vi "JV Measurement.vi"(4 "Compliance (A)":dbl=0.01, 6 "Force Channel":u16(ring) items=["Channel A", "Channel B"], 8 "Delay (s)":dbl, 9 "Max (V)":dbl, 11 "Step (V)":dbl=0.1) -> ()   [LabVIEW 2011]
uses:
  <vilib>/Utility/file.llb/Write To Spreadsheet File (string).vi
  C:/Program Files (x86)/National Instruments/LabVIEW 2009/instr.lib/Keithley 2600 Series/Keithley 2600 Series.lvlib
panel:
  in  "Sample Name":string
  in  "Device Area (cm^2)":dbl=0.12
  out "XY Graph":cluster{dbl[], dbl[]}(graph)
  in  "Experiment Title":string
  in  "User Name":string
  in  "Stabilisation level \n(A or V depending on mode)":dbl=-1.6
  in  "Stabilisation time (ms)":dbl
  in  "Stabilisation mode":u16(ring) items=["Current", "Voltage"]
  in  "Max to min voltage sweep first?":bool
  in  "Min (V)":dbl=-1.6
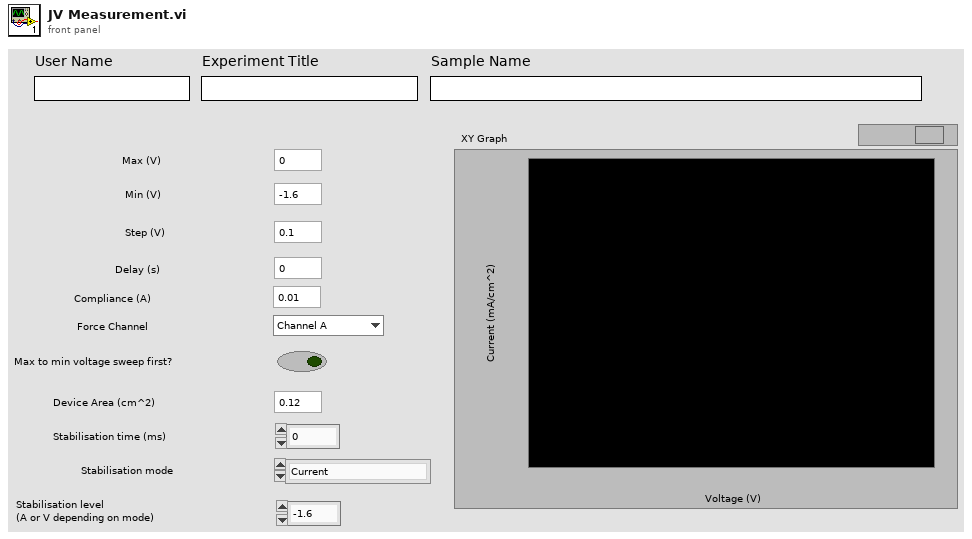
[diagram p1: front panel]
types:
  T1 = enum32{"Current", "Voltage", "IV", "Resistance", "Power"}
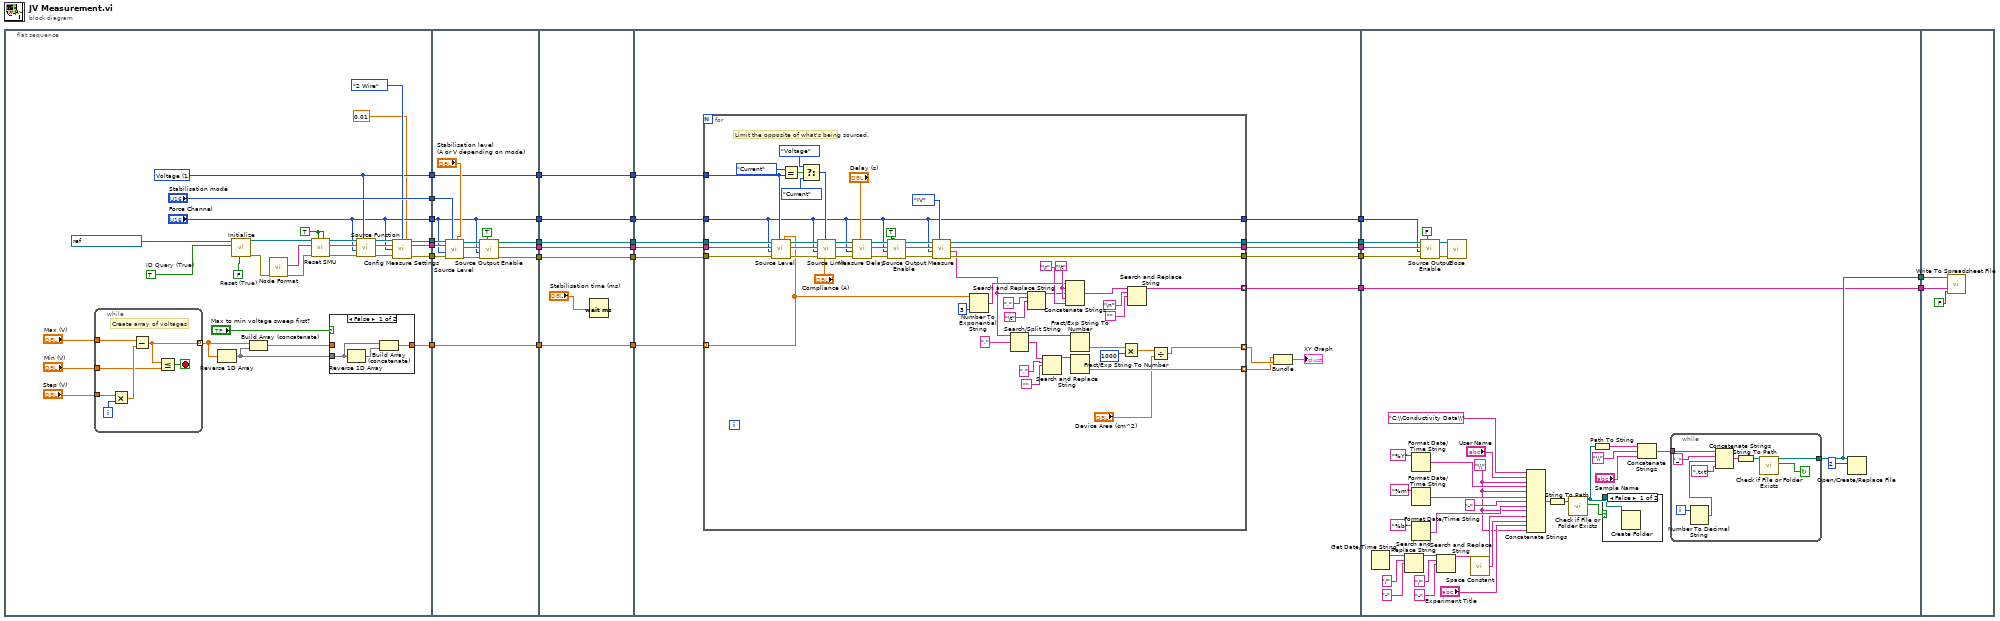
[diagram p0: block diagram]
diagram:
  n1 = flat-sequence {
    tunnel: [w29] -> w26
    tunnel: [w30] -> w25
    tunnel: ["Stabilisation mode"] -> w24
    tunnel: ["Force Channel"] -> w23
    tunnel: [w38] -> w22
    tunnel: [w37] -> w21
    tunnel: [w36] -> w20
    tunnel: w26 -> [w69]
    tunnel: w25 -> [w82]
    tunnel: w24 -> [w71]
    tunnel: w23 -> [w68]
    tunnel: w22 -> [w75]
    tunnel: w21 -> [w77]
    tunnel: w20 -> [w76]
    tunnel: [w82] -> w19
    tunnel: [w74] -> w16
    tunnel: [w73] -> w14
    tunnel: [w72] -> w12
    tunnel: [w69] -> w10
    tunnel: [w68] -> w8
    tunnel: w19 -> [w89]
    tunnel: [w89] -> w18
    tunnel: [w88] -> w17
    tunnel: w16 -> [w88]
    tunnel: [w87] -> w15
    tunnel: w14 -> [w87]
    tunnel: [w86] -> w13
    tunnel: w12 -> [w86]
    tunnel: [w84] -> w11
    tunnel: w10 -> [w84]
    tunnel: [w83] -> w9
    tunnel: w8 -> [w83]
    tunnel: w18 -> [w100]
    tunnel: w17 -> [w103]
    tunnel: w15 -> [w102]
    tunnel: w13 -> [w101]
    tunnel: w11 -> [w99]
    tunnel: w9 -> [w98]
    tunnel: [w97] -> w7
    tunnel: [w96] -> w6
    tunnel: [w95] -> w5
    tunnel: [w94] -> w4
    tunnel: [w93] -> w3
    tunnel: w7 -> [w158]
    tunnel: w6 -> [w193]
    tunnel: w5 -> [w192]
    tunnel: w4 -> [w191]
    tunnel: w3 -> [w190]
    tunnel: [w159] -> w2
    tunnel: [w158] -> w1
    tunnel: w2 -> [w206]
    tunnel: w1 -> [w205]
    frame #0 {
      w40 = TRUE
      w32 = FALSE  # Reset (True)
      w49 = TRUE  # ID Query (True)
      w29 = u16 1 items=["Current", "Voltage"] ("Source Function")
      n2 = while {
        tunnel: "Max (V)" -> [w67]
        tunnel: "Step (V)" -> [w66]
        tunnel: "Min (V)" -> [w63]
        tunnel: [w61] -> w31 mode=indexing
        i -> [w65]
        stop <- w62 stop-if-true
        # "Create array of voltages"
        n3 = Multiply(x=w66, y=w65) -> (x*y=w64:dbl)
        n4 = Subtract(x=w67, y=w64) -> (x-y=w61:dbl)
        n5 = Less Or Equal?(x=w61, y=w63) -> (x <= y?=w62:bool)
      }
      n6 = Reverse 1D Array(array=w31) -> (reversed array=w51:dbl[])
      n7 = call "Initialize.vi"("Reset (True)"=w32, "ID Query (True)"=w49, "VISA resource name"=refnum<visa-resource-name> "GPIB0::26::INSTR") -> ("error out"=w44:errorcluster, "VISA resource name out"=w42:refnum<visa-resource-name>)  [unwired: 3 in, 4 out]
      n8 = Build Array (concatenate)(w31, w51) -> (w52:dbl[])
      n9 = call "Node Format.vi"("error in"=w44) -> ("error out"=w43:errorcluster, "Formatted Node"=w45:string)  [unwired: 1 in, 8 out]
      n10 = call "Reset SMU.vi"("SMU B (No)"=w40, "SMU A (No)"=w40, "error in (no error)"=w43, "Node In"=w45, "VISA resource name"=w42) -> ("error out"=w48:errorcluster, "Node Out"=w46:string, "VISA resource name out"=w47:refnum<visa-resource-name>)  [unwired: 4 out]
      n11 = case shown="False" "Max to min voltage sweep first?" {
        tunnel: [w58 w60] -> w30
        tunnel: w52 -> [_ w60]
        tunnel: w51 -> [w59 _]
        frame False {
          n12 = Reverse 1D Array(array=w59) -> (reversed array=w57:dbl[])
          n13 = Build Array (concatenate)(w59, w57) -> (w58:dbl[])
        }
        frame True {
        }
      }
      n14 = call "Source Function.vi"("Function (Current)"=w29, "error in (no error)"=w48, "Channel (Channel A)"="Force Channel", "Node In"=w46, "VISA resource name"=w47) -> ("error out"=w34:errorcluster, "Node Out"=w41:string, "VISA resource name out"=w35:refnum<visa-resource-name>)  [unwired: 4 out]
      n15 = call "Config Measure Settings.vi"("VISA resource name"=w35, "Sense (2 Wire)"=enum32{"2 Wire", "4 Wire"}."2 Wire" ("x"), "NPLC (1.000)"=0.01, "Node In"=w41, "Channel (Channel A)"="Force Channel", "error in"=w34) -> ("VISA resource name out"=w37:refnum<visa-resource-name>, "Node Out"=w36:string, "error out"=w38:errorcluster)  [unwired: 6 in, 1 out]
    }
    frame #1 {
      n16 = call "Source Level.vi"("Level (0.000)"="Stabilisation level \n(A or V depending on mode)", "Function (Current)"=w71, "error in (no error)"=w75, "Channel (Channel A)"=w68, "Node In"=w76, "VISA resource name"=w77) -> ("error out"=w81:errorcluster, "Node Out"=w80:string, "VISA resource name out"=w79:refnum<visa-resource-name>)  [unwired: 3 out]
      n17 = call "Source Output Enable.vi"("Output (Off)"=TRUE, "error in (no error)"=w81, "Channel (Channel A)"=w68, "Node In"=w80, "VISA resource name"=w79) -> ("error out"=w72:errorcluster, "Node Out"=w73:string, "VISA resource name out"=w74:refnum<visa-resource-name>)  [unwired: 4 out]
    }
    frame #2 {
      n18 = Wait (ms)(milliseconds to wait="Stabilisation time (ms)") -> ()  [unwired: 1 out]
    }
    frame #3 {
      n19 = for {
        tunnel: w99 -> [w150]
        tunnel: w103 -> [w142]
        tunnel: w102 -> [w141]
        tunnel: w101 -> [w140]
        tunnel: w98 -> [w110]
        tunnel: [w133] -> w96
        tunnel: [w132] -> w95
        tunnel: [w131] -> w94
        tunnel: [w126] -> w90 mode=indexing
        tunnel: [w104] -> w91 mode=indexing
        tunnel: w100 -> [w109] mode=indexing
        tunnel: [w111] -> w97 mode=indexing
        tunnel: [w110] -> w93
        w137 = "\t"
        # "Limit the opposite of what's being sourced."
        n20 = call "Source Level.vi"("Level (0.000)"=w109, "Function (Current)"=w150, "error in (no error)"=w140, "Channel (Channel A)"=w110, "Node In"=w141, "VISA resource name"=w142) -> ("error out"=w157:errorcluster, "Node Out"=w152:string, "VISA resource name out"=w156:refnum<visa-resource-name>)  [unwired: 3 out]
        n21 = Equal?(x=enum32{"Current", "Voltage"}."Current", y=w150) -> (x = y?=w148:bool)
        n22 = Select(t=enum32{"Current", "Voltage"}."Voltage" ("x"), s=w148, f=enum32{"Current", "Voltage"}."Current") -> (s? t:f=w146:enum32{"Current", "Voltage"})
        n23 = call "Source Limit.vi"("Limit (0.000)"="Compliance (A)", "Function (Current)"=w146, "error in (no error)"=w157, "Channel (Channel A)"=w110, "Node In"=w152, "VISA resource name"=w156) -> ("error out"=w115:errorcluster, "Node Out"=w116:string, "VISA resource name out"=w118:refnum<visa-resource-name>)  [unwired: 3 out]
        n24 = call "Measure Delay.vi"("Delay (0)"="Delay (s)", "error in (no error)"=w115, "Channel (Channel A)"=w110, "Node In"=w116, "VISA resource name"=w118) -> ("error out"=w113:errorcluster, "Node Out"=w114:string, "VISA resource name out"=w117:refnum<visa-resource-name>)  [unwired: 3 in, 1 out]
        n25 = call "Source Output Enable.vi"("Output (Off)"=TRUE, "error in (no error)"=w113, "Channel (Channel A)"=w110, "Node In"=w114, "VISA resource name"=w117) -> ("error out"=w155:errorcluster, "Node Out"=w151:string, "VISA resource name out"=w154:refnum<visa-resource-name>)  [unwired: 4 out]
        n26 = call "Measure.vi"("Function (Current)"=T1."IV" ("Measure Function"), "error in (no error)"=w155, "Channel (Channel A)"=w110, "Node In"=w151, "VISA resource name"=w154) -> ("error out"=w131:errorcluster, "Output"=w125:string, "Node Out"=w132:string, "VISA resource name out"=w133:refnum<visa-resource-name>)  [unwired: 2 in, 1 out]
        n27 = Number To Exponential String(number=w109, precision (6)=3) -> (E-format string=w134:string)  [unwired: 2 in]
        n28 = Search/Split String(string=w125, search string/char (-)=",") -> (substring before match=w124:string, match + rest of string=w121:string)  [unwired: 1 in, 1 out]
        n29 = Search and Replace String(input string=w125, search string=",", replace string="\t") -> (result string=w127:string)  [unwired: 5 in, 3 out]
        n30 = Search and Replace String(input string=w121, search string=",", replace string="") -> (result string=w122:string)  [unwired: 5 in, 3 out]
        n31 = Concatenate Strings(w134, w137, w127, w137, "\r") -> (w139:string)
        n32 = Fract/Exp String To Number(string=w124) -> (number=w108:dbl)  [unwired: 3 in, 1 out]
        n33 = Fract/Exp String To Number(string=w122) -> (number=w126:dbl)  [unwired: 3 in, 1 out]
        n34 = Multiply(x=w108, y=1000) -> (x*y=w107:dbl)
        n35 = Search and Replace String(input string=w139, search string="\n", replace string="") -> (result string=w111:string)  [unwired: 5 in, 3 out]
        n36 = Divide(x=w107, y="Device Area (cm^2)") -> (x/y=w104:dbl)
      }
      n37 = Bundle(w90, w91) -> (→"XY Graph":cluster{dbl[], dbl[]})  [unwired: 1 in]
    }
    frame #4 {
      w169 = "\\"
      n38 = Get Date/Time String() -> (date string=w178:string)  [unwired: 3 in, 1 out]
      n39 = Search and Replace String(input string=w178, search string="/", replace string="-") -> (result string=w173:string)  [unwired: 5 in, 3 out]
      n40 = Format Date/Time String(time format string (%c)="%Y") -> (date/time string=w182:string)  [unwired: 2 in]
      n41 = Format Date/Time String(time format string (%c)="%m") -> (date/time string=w181:string)  [unwired: 2 in]
      n42 = Format Date/Time String(time format string (%c)="%b") -> (date/time string=w180:string)  [unwired: 2 in]
      n43 = call "Source Output Enable.vi"("Output (Off)"=FALSE, "error in (no error)"=w191, "Channel (Channel A)"=w190, "Node In"=w192, "VISA resource name"=w193) -> ("error out"=w188:errorcluster, "VISA resource name out"=w189:refnum<visa-resource-name>)  [unwired: 5 out]
      n44 = Search and Replace String(input string=w173, search string="/", replace string="-") -> (result string=w172:string)  [unwired: 5 in, 3 out]
      n45 = call "Close.vi"("error in (no error)"=w188, "VISA resource name"=w189) -> ()  [unwired: 10 out]
      n46 = call <vilib>:"Space Constant.vi"() -> ("String"=w171:string)
      n47 = Concatenate Strings("C:\\Conductivity Data\\", "User Name", w169, w182, w169, w181, "-", w180, w169, w172, w171, "Experiment Title", w169) -> (w162:string)
      n48 = String To Path(string=w162) -> (path=w161:path)
      n49 = call <vilib>:"Check if File or Folder Exists.vi"("path"=w161) -> ("file or folder exists?"=w165:bool, "dup path"=w167:path)  [unwired: 8 in, 1 out]
      n50 = Path To String(path=w167) -> (string=w166:string)
      n51 = case shown="False" w165 {
        tunnel: w167 -> [w195 _]
        frame False {
          n52 = Create Folder(path (use dialog)=w195) -> ()  [unwired: 2 in, 3 out]
        }
        frame True {
        }
      }
      n53 = Concatenate Strings(w166, "\\", "Sample Name") -> (w160:string)
      n54 = while {
        tunnel: w160 -> [w204]
        tunnel: [w196] -> w159
        i -> [w202]
        stop <- w197 continue-if-true
        n55 = Number To Decimal String(number=w202) -> (decimal integer string=w201:string)  [unwired: 1 in]
        n56 = Concatenate Strings(w204, "_", w201, ".txt") -> (w198:string)
        n57 = String To Path(string=w198) -> (path=w199:path)
        n58 = call <vilib>:"Check if File or Folder Exists.vi"("path"=w199) -> ("file or folder exists?"=w197:bool, "dup path"=w196:path)  [unwired: 8 in, 1 out]
      }
      n59 = Open/Create/Replace File(file path (use dialog)=w159, operation (0:open)=2) -> ()  [unwired: 4 in, 3 out]
    }
    frame #5 {
      n60 = call-poly <vilib>:"Write To Spreadsheet File.vi"("append to file? (new file:F)"=FALSE, "1D data"=w205, "file path (dialog if empty)"=w206) -> ()  [unwired: 5 in, 1 out]
    }
  }
